vi "SVL Send Data to Waterfall.vi"   [LabVIEW 2017]
doc: "Sends the waterfall data to the waterfall display. You can use this polymorphic VI to send waterfall data to the waterfall display using a 2D array or a cluster. The data type you wire to the <B>waterfall data</B> input determines the polymorphic instance to use."
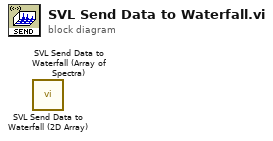
[diagram p0: block diagram]
diagram:
  n1 = call <vilib>:"SVL Send Data to Waterfall (2D Array).vi"() -> ()  [unwired: 14 in, 2 out]
  n2 = call <vilib>:"SVL Send Data to Waterfall (Array of Spectra).vi"() -> ()  [unwired: 14 in, 2 out]
